vi "fxpPositionControls.vi"(9 "visibleOverflowStatus":bool, 10 "visibleModes":bool, 11 "fxpXctl refnums":T1) -> ()   [LabVIEW 2017, in "FXP.xctl"]
uses:
  <vilib>/fxp/FXPxcontrol/FXP.xctl
  <vilib>/fxp/FXPxcontrol/fxpFacadeCtlRefnums.ctl
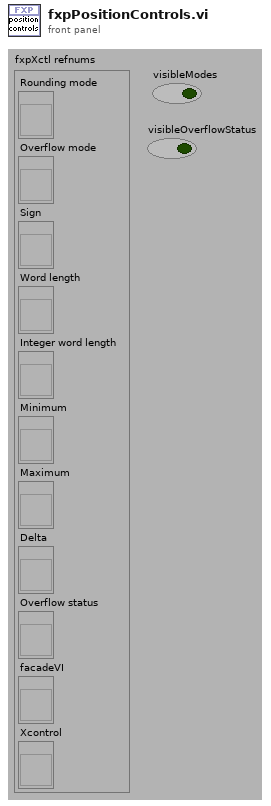
[diagram p1: front panel]
types:
  T1 = typedef "FXP.xctl/fxpFacadeCtlRefnums.ctl" = cluster{"Rounding mode":refnum<vi>, "Overflow mode":refnum<vi>, "Sign":refnum<vi>, "Word length":refnum<vi>, "Integer word length":refnum<vi>, "Minimum":refnum<vi>, "Maximum":refnum<vi>, "Delta":refnum<vi>, "Overflow status":refnum<vi>, "facadeVI":refnum<vi>, "Xcontrol":refnum<vi>}
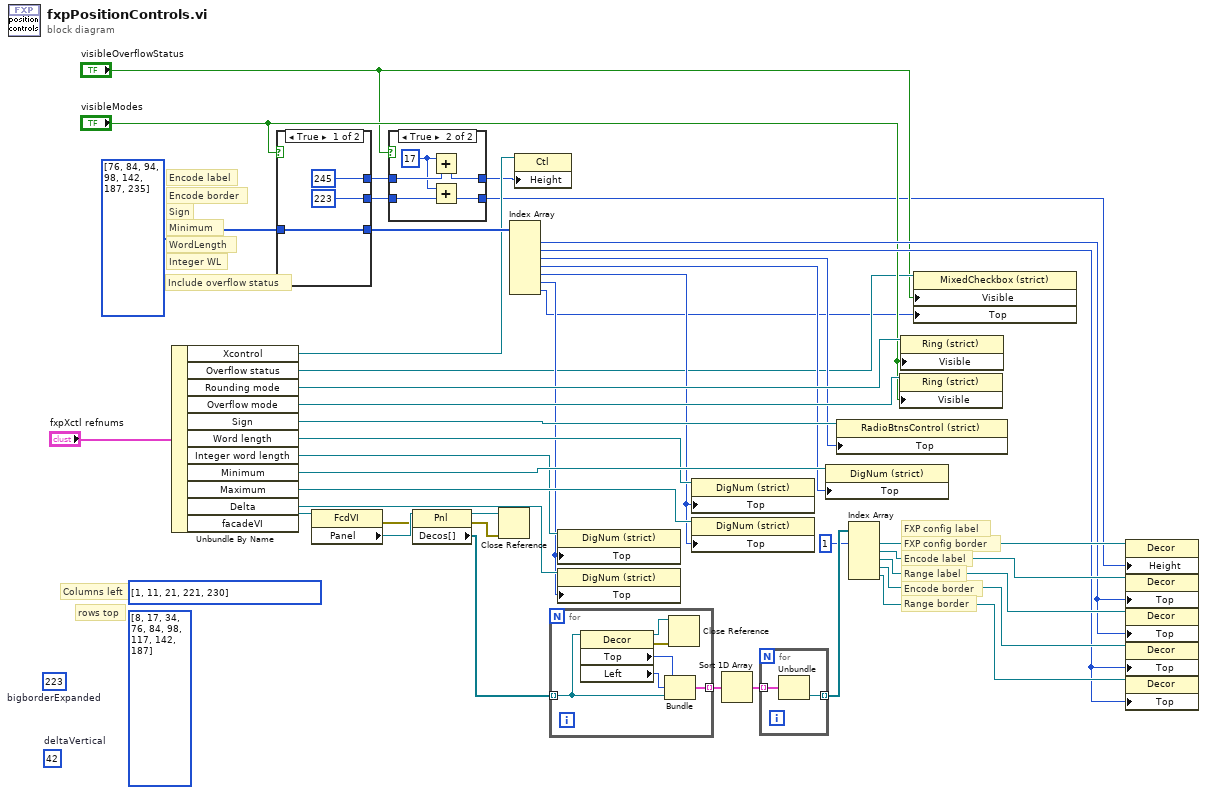
[diagram p0: block diagram]
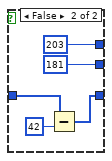
[diagram p3: hidden frame]
diagram:
  (unwired) 42  # deltaVertical
  (unwired) i32[] [8, 17, 34, 76, 84, 98, 117, 142, 187]
  (unwired) i32[] [1, 11, 21, 221, 230]
  (unwired) 223  # bigborderExpanded
  # "Include overflow status"
  # "Integer WL"
  # "WordLength"
  # "Minimum"
  # "Sign"
  # "Encode border"
  # "Encode label"
  # "Range border"
  # "Encode border"
  # "Range label"
  # "Encode label"
  # "FXP config border"
  # "FXP config label"
  # "rows top"
  # "Columns left"
  n1 = Unbundle By Name("fxpXctl refnums") -> ("Xcontrol"=w11:refnum<vi>, "Overflow status"=w7:refnum<vi>, "Rounding mode"=w31:refnum<vi>, "Overflow mode"=w30:refnum<vi>, "Sign"=w29:refnum<vi>, "Word length"=w27:refnum<vi>, "Integer word length"=w25:refnum<vi>, "Minimum"=w28:refnum<vi>, "Maximum"=w26:refnum<vi>, "Delta"=w24:refnum<vi>, "facadeVI"=w13:refnum<vi>)
  n2 = case shown="True" "visibleModes" {
    tunnel: [u32 223 ("Size:Height") u32 181 ("Size:Height")] -> w3
    tunnel: [w43 w46] -> w23
    tunnel: i32[] [76, 84, 94, 98, 142, 187, 235] -> [w43 w47]
    tunnel: [u32 245 ("Size:Height") u32 203 ("Size:Height")] -> w5
    frame True {
    }
    frame False {
      n3 = Subtract(x=w47, y=42 ("Size:Height")) -> (x-y=w46:i32[])
    }
  }
  n4 = property class="FcdVI"(reference=w13) -> (error out=w14:errorcluster, "Panel"=w15:refnum<vi>)  [unwired: 1 in, 1 out]
  n5 = case shown="True" "visibleOverflowStatus" {
    tunnel: w5 -> [w51 w56]
    tunnel: [w51 w55] -> w4
    tunnel: [w50 w53] -> w2
    tunnel: w3 -> [w50 w54]
    frame False {
    }
    frame True {
      w52 = u32 17 ("x")
      n6 = Add(x=w52, y=w56) -> (x+y=w55:u32)
      n7 = Add(x=w52, y=w54) -> (x+y=w53:u32)
    }
  }
  n8 = property class="Pnl"(reference=w15, error in=w14) -> (reference out=w9:refnum<vi>, error out=w10:errorcluster, "Decos[]"=w12:refnum<vi>[])
  n9 = Close Reference(reference=w9, error in (no error)=w10) -> ()  [unwired: 1 out]
  n10 = Index Array(array=w23) -> (element #1=w21:i32, element #2=w20:i32, element #3=w19:i32, element #4=w8:i32, element #5=w18:i32, element #6=w17:i32, element #7=w1:i32)  [unwired: 7 in]
  n11 = property class="Ctl"(reference=w11, "Height"=w4) -> ()  [unwired: 1 in, 2 out]
  n12 = for {
    tunnel: w12 -> [w62] mode=indexing
    tunnel: [w59] -> w40 mode=indexing
    n13 = property class="Decor"(reference=w62) -> (reference out=w57:refnum<vi>, error out=w58:errorcluster, "Top"=w61:i32, "Left"=w60:i32)  [unwired: 1 in]
    n14 = Bundle("Top"=w61, "Left"=w60, w62) -> (w59:cluster{"Top":i32, "Left":i32, refnum<vi>})  [unwired: 1 in]
    n15 = Close Reference(reference=w57, error in (no error)=w58) -> ()  [unwired: 1 out]
  }
  n16 = property class="DigNum (strict)"(reference=w25, "Top"=w17) -> ()  [unwired: 1 in, 2 out]
  n17 = property class="DigNum (strict)"(reference=w24, "Top"=w17) -> ()  [unwired: 1 in, 2 out]
  n18 = property class="DigNum (strict)"(reference=w27, "Top"=w18) -> ()  [unwired: 1 in, 2 out]
  n19 = property class="DigNum (strict)"(reference=w26, "Top"=w18) -> ()  [unwired: 1 in, 2 out]
  n20 = Sort 1D Array(array=w40) -> (sorted array=w39:cluster{"Top":i32, "Left":i32, refnum<vi>}[])
  n21 = for {
    tunnel: w39 -> [w64] mode=indexing
    tunnel: [w63] -> w38 mode=indexing
    n22 = Unbundle(w64) -> (w63:refnum<vi>)  [unwired: 2 out]
  }
  n23 = property class="DigNum (strict)"(reference=w28, "Top"=w8) -> ()  [unwired: 1 in, 2 out]
  n24 = property class="RadioBtnsControl (strict)"(reference=w29, "Top"=w19) -> ()  [unwired: 1 in, 2 out]
  n25 = Index Array(array=w38, index #1=1 ("index")) -> (element #1=w36:refnum<vi>, element #2=w35:refnum<vi>, element #3=w34:refnum<vi>, element #4=w33:refnum<vi>, element #5=w32:refnum<vi>)  [unwired: 4 in]
  n26 = property class="Ring (strict)"(reference=w30, "Visible"="visibleModes") -> ()  [unwired: 1 in, 2 out]
  n27 = property class="Ring (strict)"(reference=w31, "Visible"="visibleModes") -> ()  [unwired: 1 in, 2 out]
  n28 = property class="MixedCheckbox (strict)"(reference=w7, "Visible"="visibleOverflowStatus", "Top"=w1) -> ()  [unwired: 1 in, 2 out]
  n29 = property class="Decor"(reference=w36, "Height"=w2) -> ()  [unwired: 1 in, 2 out]
  n30 = property class="Decor"(reference=w35, "Top"=w21) -> ()  [unwired: 1 in, 2 out]
  n31 = property class="Decor"(reference=w34, "Top"=w21) -> ()  [unwired: 1 in, 2 out]
  n32 = property class="Decor"(reference=w33, "Top"=w20) -> ()  [unwired: 1 in, 2 out]
  n33 = property class="Decor"(reference=w32, "Top"=w20) -> ()  [unwired: 1 in, 2 out]
